vi "Manager Icon.vi"() -> (3 "Manager Icon":picture)   [LabVIEW 2020, in "Parallel Diagram Block.xnode"]
uses:
  Parallel Diagram Block.xnode
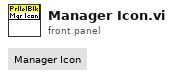
[diagram p1: front panel]
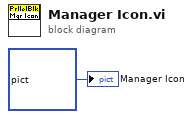
[diagram p0: block diagram]
diagram:
  "Manager Icon" <- picture bytes[12830] ("2D Picture")
